vi "Apend Test Case Result.vi"(8 "error in (no error)":errorcluster, 9 "Test Case Result":T1, 11 "Plain Text Report In":refnum<class "Plain Text Report.lvclass">) -> (0 "error out":errorcluster, 3 "Plain Text Report Out":refnum<class "Plain Text Report.lvclass">)   [LabVIEW 2020, in "Plain Text Report.lvclass"]
uses:
  Plain Text Report.lvclass
  Result Types/Case Result/Test Case Result.ctl
  Result Types/Method Result/Method Result.ctl
  Rewrite Project/Result/Status.ctl
  Result Types/Assertion Result/Assertion Result.ctl
  Result Types/Assertion Result/Public/TypeDefs/Assertion Type.ctl
  Plain Text Report.lvclass/Plain Text Report.ctl
  Result Types/Case Result/Test Case Result.lvlib
  Result Types/Assertion Result/Assertion Result.lvlib
  Result Types/Method Result/Method Result.lvlib
  Rewrite Project/Result/Result.lvlib
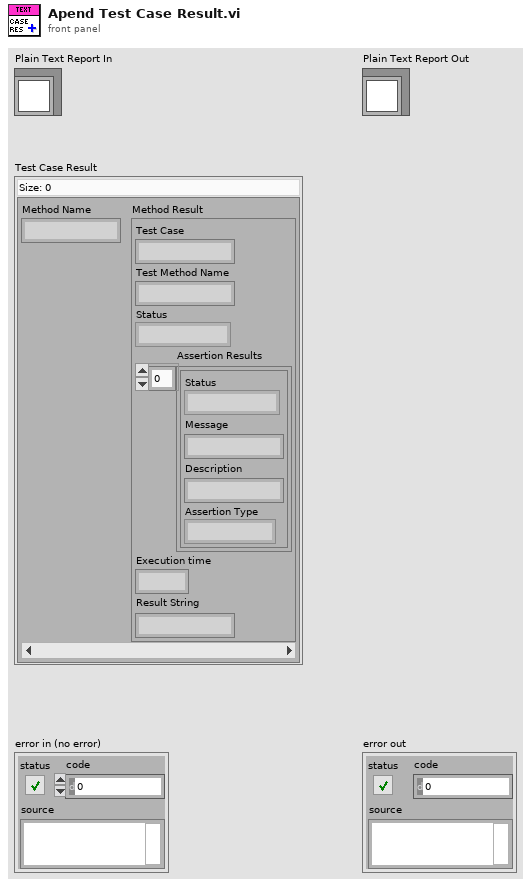
[diagram p1: front panel]
types:
  T1 = typedef "Test Case Result.lvlib/Test Case Result.ctl" = map{string, T2}
  T2 = typedef "Method Result.lvlib/Method Result.ctl" = cluster{"Test Case":string, "Test Method Name":string, "Status":T3, "Assertion Results":T4[], "Execution time":dbl, "Result String":string}
  T3 = typedef "Result.lvlib/Status.ctl" = enum16{"Pass", "Fail", "Error", "Skipped", "Setup Error", "Broken", "Teardown Error"}
  T4 = typedef "Assertion Result.lvlib/Assertion Result.ctl" = cluster{"Status":T3, "Message":string, "Description":string, "Assertion Type":T5}
  T5 = typedef "Result.lvlib/Assertion Type.ctl" = enum16{"None", "Pass", "Fail", "Skip", "Pass if Equal", "Fail if Equal", "Pass if Error", "Fail if Error", "Pass if", "Fail if"}
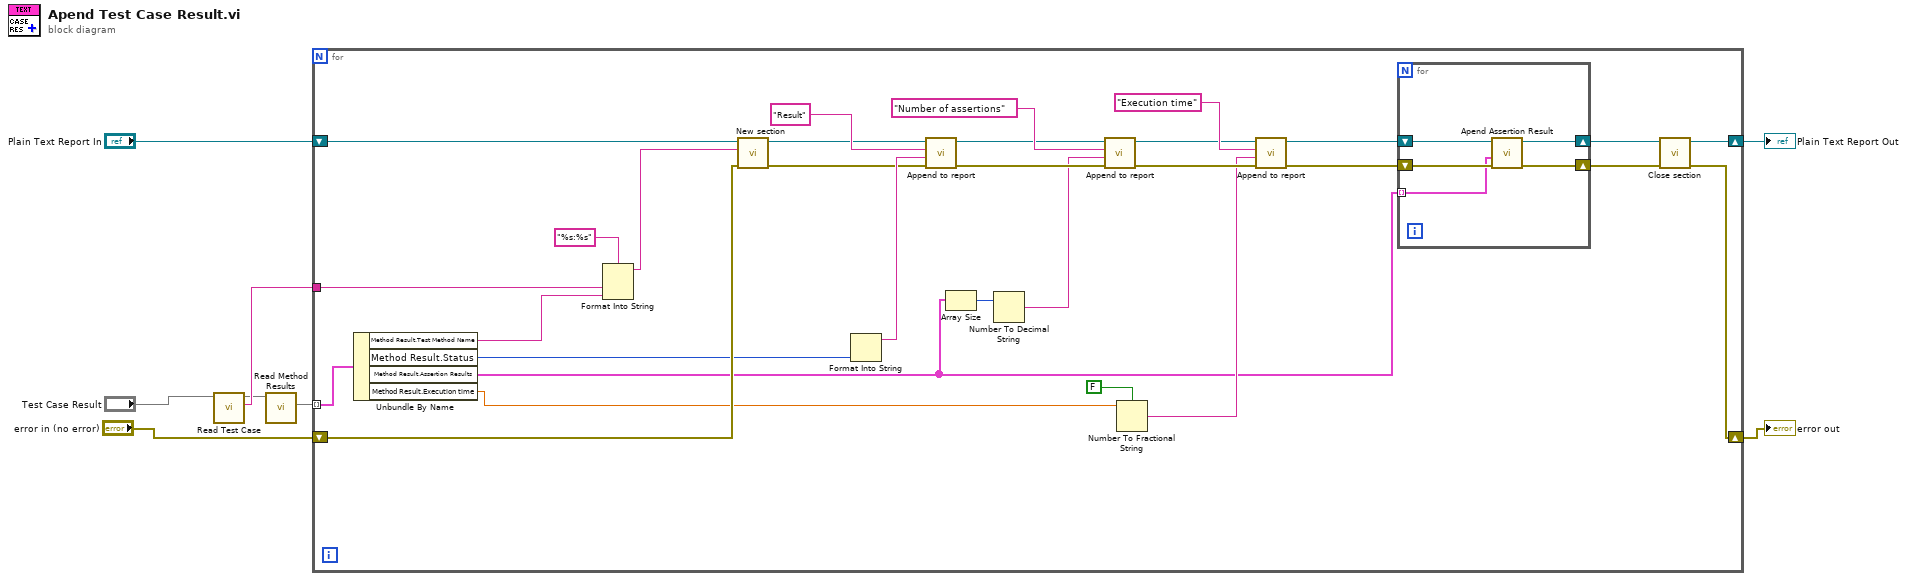
[diagram p0: block diagram]
diagram:
  n1 = call "Read Test Case.vi"("Test Case Result In"="Test Case Result") -> ("Test Case"=w5:string, "Test Case Result Out"=w4:T1)  [unwired: 9 in]
  n2 = call "Read Method Results.vi"("Test Case Result In"=w4) -> ("Method Results"=w3:map{string, T2})  [unwired: 9 in, 1 out]
  n3 = for {
    shift-right: [w25] -> w7
    shift-left: "Plain Text Report In" -> [w35]
    tunnel: w5 -> [w37]
    tunnel: w3 -> [w12] mode=indexing
    shift-right: [w23] -> w2
    shift-left: "error in (no error)" -> [w22]
    n4 = Unbundle By Name(w12) -> ("Method Result.Test Method Name"=w17:string, "Method Result.Status"=w16:T3, "Method Result.Assertion Results"=w9:T4[], "Method Result.Execution time"=w11:dbl)
    n5 = Format Into String(format string="%s:%s", w37, w17) -> (resulting string=w36:string)  [unwired: 2 in, 1 out]
    n6 = call "New section.vi"("error in (no error)"=w22, "Section name"=w36, "Plain Text Report In"=w35) -> ("error out"=w21:errorcluster, "Plain Text Report Out"=w31:refnum<class "Plain Text Report.lvclass">)  [unwired: 7 in]
    n7 = Format Into String(w16) -> (resulting string=w32:string)  [unwired: 3 in, 1 out]
    n8 = call "Append to report.vi"("error in (no error)"=w21, "Value"=w32, "Key"="Result" ("Name"), "Plain Text Report In"=w31) -> ("error out"=w20:errorcluster, "Plain Text Report Out"=w29:refnum<class "Plain Text Report.lvclass">)  [unwired: 6 in]
    n9 = Array Size(array=w9) -> (size(s)=w15:i32)
    n10 = Number To Decimal String(number=w15) -> (decimal integer string=w14:string)  [unwired: 1 in]
    n11 = call "Append to report.vi"("error in (no error)"=w20, "Value"=w14, "Key"="Number of assertions" ("Name"), "Plain Text Report In"=w29) -> ("error out"=w19:errorcluster, "Plain Text Report Out"=w28:refnum<class "Plain Text Report.lvclass">)  [unwired: 6 in]
    n12 = Number To Fractional String(use system decimal point (T)=FALSE, number=w11) -> (F-format string=w10:string)  [unwired: 2 in]
    n13 = call "Append to report.vi"("error in (no error)"=w19, "Value"=w10, "Key"="Execution time" ("Name"), "Plain Text Report In"=w28) -> ("error out"=w18:errorcluster, "Plain Text Report Out"=w27:refnum<class "Plain Text Report.lvclass">)  [unwired: 6 in]
    n14 = for {
      shift-right: [w41] -> w26
      shift-left: w27 -> [w42]
      shift-right: [w43] -> w24
      shift-left: w18 -> [w40]
      tunnel: w9 -> [w39] mode=indexing
      n15 = call "Apend Assertion Result.vi"("error in (no error)"=w40, "Assertion Result"=w39, "Plain Text Report In"=w42) -> ("error out"=w43:errorcluster, "Plain Text Report Out"=w41:refnum<class "Plain Text Report.lvclass">)  [unwired: 7 in]
    }
    n16 = call "Close section.vi"("error in (no error)"=w24, "Plain Text Report In"=w26) -> ("error out"=w23:errorcluster, "Plain Text Report Out"=w25:refnum<class "Plain Text Report.lvclass">)  [unwired: 8 in]
  }
  "error out" <- w2
  "Plain Text Report Out" <- w7
